vi "test.vi"() -> ()   [LabVIEW 2019, in "MD4Logger Engine.lvlib"]
uses:
  MD4Logger Engine.lvlib
panel:
  out "Error Out 3":errorcluster
  in  "Path":path=path "C:/Users/Hovhannes/Desktop/MD4Logger/Source/Engine/DLL/WriterExample.dll"
  out "Error Out 2":errorcluster
  out "Array":u32[](array[numeric])
  out "Error Out":errorcluster
  in  "Data":u64=5
  in  "Number of Samples per Read":u32=10000
  in  "Iterations":u32=10000
  in  "MDF4 File Path":path=path "C:/Users/Hovhannes/Desktop/MDF4API/aaa.mf4"
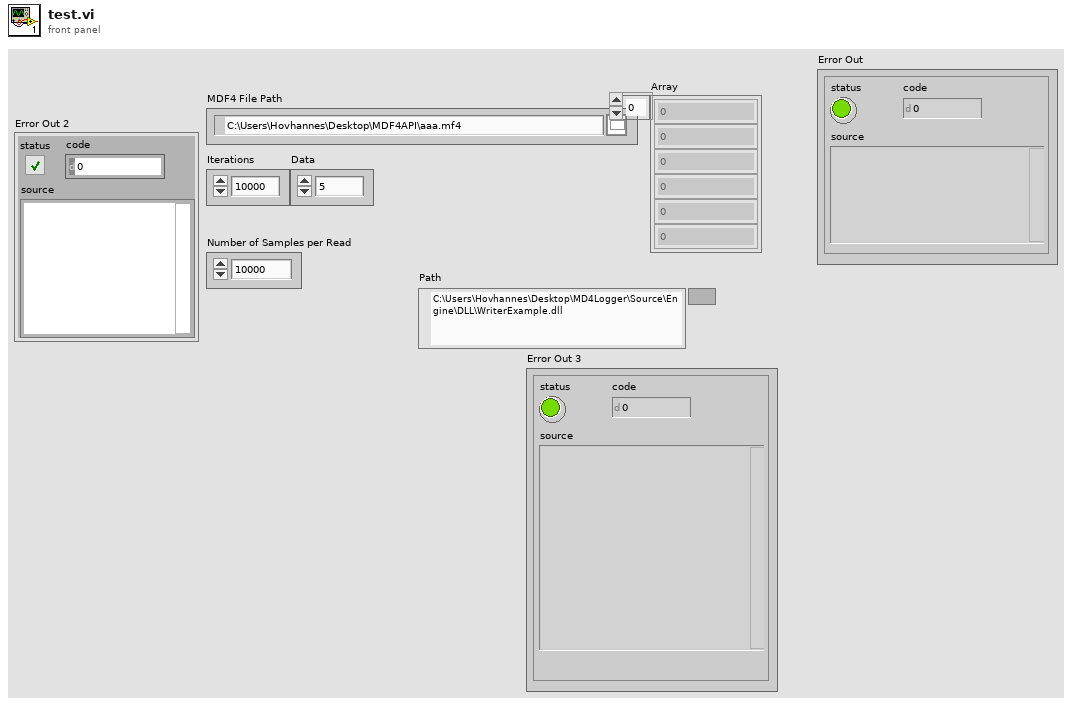
[diagram p1: front panel]
types:
  T1 = cluster{"Comment":string, "Time Source":string, "Author":string, "Department":string, "Project":string, "Subject":string}
  T2 = cluster{"History":string, "ID":string, "Vendor":string, "Version":string}
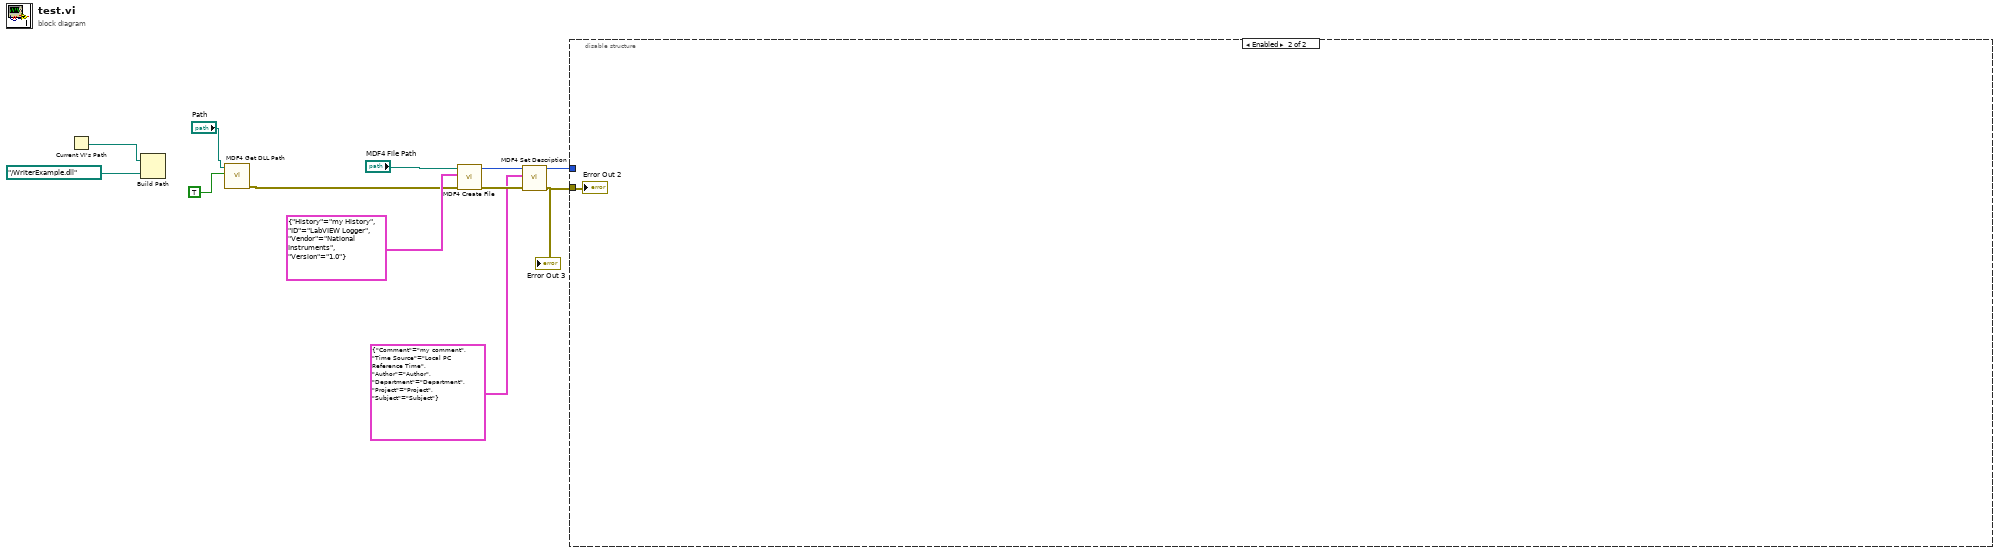
[diagram p0: block diagram]
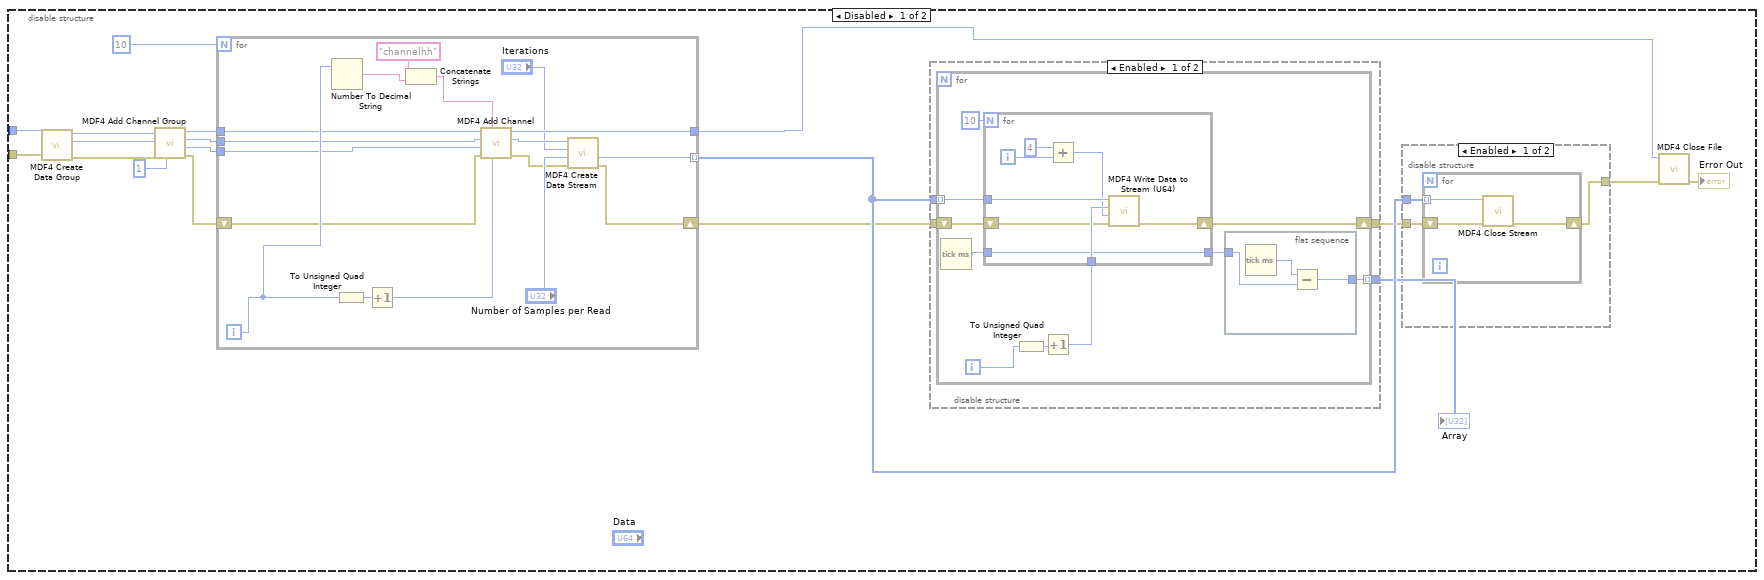
[diagram p2: hidden frame]
diagram:
  n1 = Current VI's Path() -> (path=w3:path)
  n2 = Build Path(base path=w3, name or relative path=path "../WriterExample.dll") -> ()  [unwired: 1 out]
  n3 = call "MDF4 Get DLL Path.vi"("Init"=TRUE, "DLL Path"="Path") -> ("error out"=w4:errorcluster)  [unwired: 8 in, 1 out]
  n4 = call "MDF4 Create File.vi"("Error In"=w4, "History"=T2 {"History"="my History", "ID"="LabVIEW Logger", "Vendor"="National Instruments", "Version"="1.0"}, "MDF4 File Path"="MDF4 File Path") -> ("Error Out"=w10:errorcluster, "MDF4 File Reference out"=w11:i64)  [unwired: 6 in]
  "Error Out 3" <- w10
  n5 = call "MDF4 Set Description.vi"("Error In"=w10, "Comment"=T1 {"Comment"="my comment", "Time Source"="Local PC Reference Time", "Author"="Author", "Department"="Department", "Project"="Project", "Subject"="Subject"}, "MDF4 File Reference in"=w11) -> ("Error Out"=w9:errorcluster, "MDF4 File Reference out"=w8:i64)  [unwired: 7 in]
  n6 = disable-structure shown="Enabled" {
    disable-tunnel: w9 -> [w23 w81]
    disable-tunnel: w8 -> [w22 _]
    frame Disabled {
      n7 = call "MDF4 Create Data Group.vi"("Error In"=w23, "MDF4 File Reference in"=w22) -> ("Error Out"=w21:errorcluster, "Data Group Reference out"=w20:i64, "MDF4 File Reference out"=w19:i64)  [unwired: 7 in]
      n8 = call "MDF4 Add Channel Group.vi"("Record ID"=u64 1, "Error In"=w21, "Data Group Reference in"=w20, "MDF4 File Reference in"=w19) -> ("Error Out"=w18:errorcluster, "Channel Group Reference out"=w15:i64, "Data Group Reference out"=w16:i64, "MDF4 File Reference out"=w17:i64)  [unwired: 4 in]
      n9 = for {
        N: 10 -> [_]
        tunnel: [w54] -> w30 mode=indexing
        tunnel: [w53] -> w27
        shift-right: [w52] -> w26
        shift-left: w18 -> [w42]
        tunnel: w17 -> [w41]
        tunnel: w16 -> [w40]
        tunnel: w15 -> [w39]
        i -> [w46]
        n10 = Number To Decimal String(number=w46) -> (decimal integer string=w45:string)  [unwired: 1 in]
        n11 = To Unsigned Quad Integer(1:w46) -> (0:w51:u64)
        n12 = Increment(x=w51) -> (x+1=w38:u64)
        n13 = Concatenate Strings("channelhh" ("string"), w45) -> (w43:string)
        n14 = call "MDF4 Add Channel.vi"("Channel ID"=w38, "Channel Name"=w43, "Error In"=w42, "Channel Group Reference in"=w39, "Data Group Reference in"=w40, "MDF4 File Reference in"=w41) -> ("Error Out"=w47:errorcluster, "Data Group Reference out"=w50:i64, "MDF4 File Reference out"=w53:i64)  [unwired: 3 in]
        n15 = call "MDF4 Create Data Stream.vi"("Error In"=w47, "Number of Samples per Read"="Number of Samples per Read", "Iterations"="Iterations", "Data Group Reference in"=w50) -> ("Error Out"=w52:errorcluster, "Stream Reference out"=w54:i64)  [unwired: 5 in, 1 out]
      }
      n16 = disable-structure shown="Enabled" {
        disable-tunnel: w30 -> [w58 _]
        disable-tunnel: [w57 w80] -> w29
        disable-tunnel: w26 -> [w56 w80]
        disable-tunnel: [w55 _] -> w13
        frame Enabled {
          n17 = for {
            tunnel: w58 -> [w68] mode=indexing
            shift-right: [w64] -> w57
            shift-left: w56 -> [w63]
            tunnel: [w59] -> w55 mode=indexing
            i -> [w66]
            n18 = Tick Count (ms)() -> (millisecond timer value=w61:u32)
            n19 = To Unsigned Quad Integer(1:w66) -> (0:w67:u64)
            n20 = Increment(x=w67) -> (x+1=w65:u64)
            n21 = for {
              N: 10 -> [_]
              tunnel: w68 -> [w79]
              tunnel: w65 -> [w78]
              shift-right: [w77] -> w64
              shift-left: w63 -> [w76]
              tunnel: w61 -> [w72]
              tunnel: [w72] -> w60
              i -> [w75]
              n22 = Add(x=4, y=w75) -> (x+y=w73:i32)
              n23 = call "MDF4 Write Data to Stream (U64).vi"("Error In"=w76, "Data"=w73, "Channel Index"=w78, "Stream Reference in"=w79) -> ("Error Out"=w77:errorcluster)  [unwired: 6 in, 1 out]
            }
            n24 = flat-sequence {
              tunnel: w60 -> [w69]
              tunnel: [w71] -> w59
              frame #0 {
                n25 = Tick Count (ms)() -> (millisecond timer value=w70:u32)
                n26 = Subtract(x=w70, y=w69) -> (x-y=w71:u32)
              }
            }
          }
        }
        frame Disabled {
        }
      }
      "Array" <- w13
      n27 = disable-structure shown="Enabled" {
        disable-tunnel: w30 -> [w33 _]
        disable-tunnel: w29 -> [w32 w37]
        disable-tunnel: [w31 w37] -> w28
        frame Enabled {
          n28 = for {
            shift-right: [w35] -> w31
            shift-left: w32 -> [w36]
            tunnel: w33 -> [w34] mode=indexing
            n29 = call "MDF4 Close Stream.vi"("Error In"=w36, "Stream Reference in"=w34) -> ("Error Out"=w35:errorcluster)  [unwired: 8 in, 1 out]
          }
        }
        frame Disabled {
        }
      }
      n30 = call "MDF4 Close File.vi"("Error In"=w28, "MDF4 File Reference in"=w27) -> ("Error Out"=→"Error Out":errorcluster)  [unwired: 8 in, 1 out]
    }
    frame Enabled {
      "Error Out 2" <- w81
    }
  }
